vi "Problem 16.vi"() -> ()   [LabVIEW 2013, in "Problem 16.lvlib"]
uses:
  Problem 16.lvlib
panel:
  out "Sum of Indiv. Digits":i32
  in  "2^x":i32
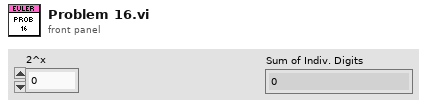
[diagram p1: front panel]
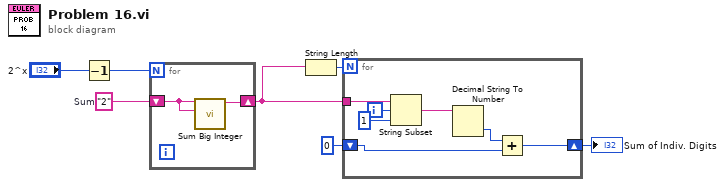
[diagram p0: block diagram]
diagram:
  w7 = "2"  # Sum
  n1 = Decrement(x="2^x") -> (x-1=w5:i32)
  n2 = for {
    N: w5 -> [_]
    shift-right: [w8] -> w3
    shift-left: w7 -> [w9]
    n3 = call "Sum Big Integer.vi"("y"=w9, "x"=w9) -> ("x+y"=w8:string)  [unwired: 9 in]
  }
  n4 = String Length(string=w3) -> (length=w4:i32)
  n5 = for {
    N: w4 -> [_]
    tunnel: w3 -> [w16]
    shift-right: [w10] -> w1
    shift-left: 0 -> [w11]
    i -> [w15]
    n6 = String Subset(string=w16, offset (0)=w15, length (rest)=1 ("length (rest)")) -> (substring=w13:string)
    n7 = Decimal String To Number(string=w13) -> (number=w12:i32)  [unwired: 2 in, 1 out]
    n8 = Add(x=w12, y=w11) -> (x+y=w10:i32)
  }
  "Sum of Indiv. Digits" <- w1
